vi "IsGet.vi"(8 "error in (no error)":errorcluster, 9 "message in":string, 11 "TCP_Server_Connection_Handler in":refnum<class "TCP_Server_Connection_Handler.lvclass">) -> (0 "error out":errorcluster, 1 "message out":string, 2 "IsGet?":bool, 3 "TCP_Server_Connection_Handler out":refnum<class "TCP_Server_Connection_Handler.lvclass">, 4 "Filename":string)   [LabVIEW 2023, in "TCP_Server_Connection_Handler.lvlib" / "TCP_Server_Connection_Handler.lvclass"]
uses:
  TCP_Server_Connection_Handler.lvclass
  TCP_Server_Connection_Handler.lvclass/TCP_Server_Connection_Handler.ctl
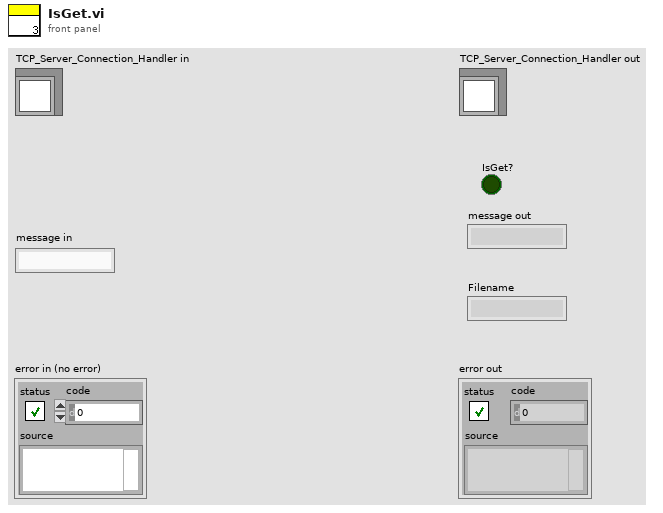
[diagram p1: front panel]
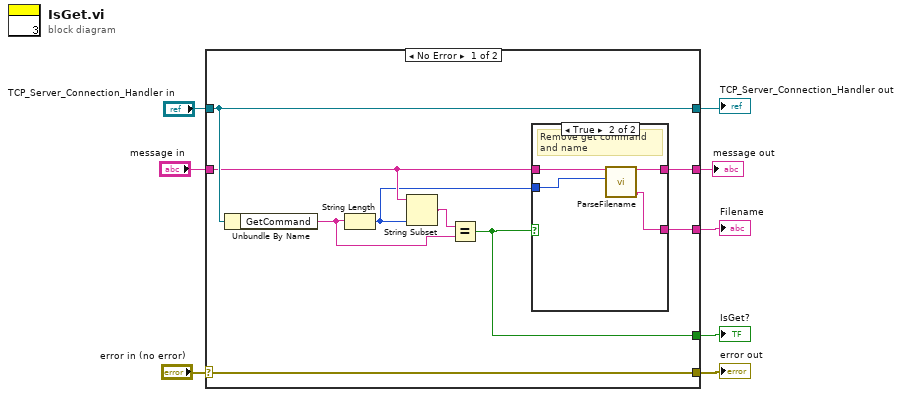
[diagram p0: block diagram]
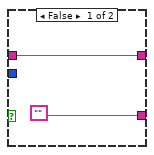
[diagram p2: hidden frame]
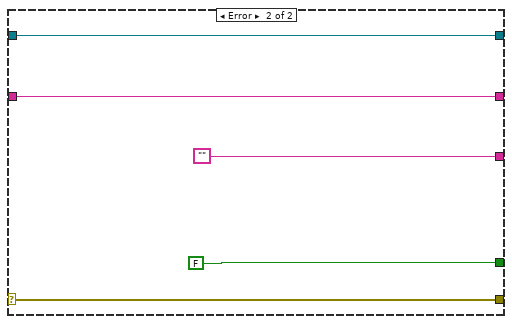
[diagram p3: hidden frame]
diagram:
  n1 = case shown="No Error" "error in (no error)" {
    selector: "error in (no error)" -> [w17 w28]
    tunnel: [w17 w28] -> w7
    tunnel: [w16 w27] -> w5
    tunnel: "TCP_Server_Connection_Handler in" -> [w16 w27]
    tunnel: [w13 FALSE] -> w4
    tunnel: "message in" -> [w12 w26]
    tunnel: [w10 w26] -> w2
    tunnel: [w9 ""] -> w1
    frame No Error {
      n2 = Unbundle By Name(w16) -> ("GetCommand"=w14:string)
      n3 = String Length(string=w14) -> (length=w11:i32)
      n4 = String Subset(string=w12, length (rest)=w11) -> (substring=w15:string)  [unwired: 1 in]
      n5 = Equal?(x=w15, y=w14) -> (x = y?=w13:bool)
      n6 = case shown="True" w13 {
        tunnel: w12 -> [w19 w23]
        tunnel: w11 -> [_ w21]
        tunnel: [w19 w22] -> w10
        tunnel: ["" w20] -> w9
        frame False {
        }
        frame True {
          # "Remove get command and name"
          n7 = call "ParseFilename.vi"("Length of marker"=w21, "message in in"=w23) -> ("Filename"=w20:string, "data out"=w22:string)  [unwired: 8 in]
        }
      }
    }
    frame Error {
    }
  }
  "error out" <- w7
  "TCP_Server_Connection_Handler out" <- w5
  "IsGet?" <- w4
  "message out" <- w2
  "Filename" <- w1
